vi "SetPwrSupAutomatic_v2.vi"(8 "error in (no error)":errorcluster, 10 "Enum":T1=enum."Control Power", 11 "HMP VISA":refnum<visa-resource-name>) -> (0 "error out":errorcluster, 3 "HMP VISA Out":refnum<visa-resource-name> caption="VISA resource name out")   [LabVIEW 2022 SP3]
doc: "This VI will command the Power Supply. Add enumerators and cases if new commands are needed"
uses:
  HMP4000 Communication/HMP4040_ChannelControlAutomatic.ctl
  HMP4000 Communication/HMP4040_ChannelControl.ctl
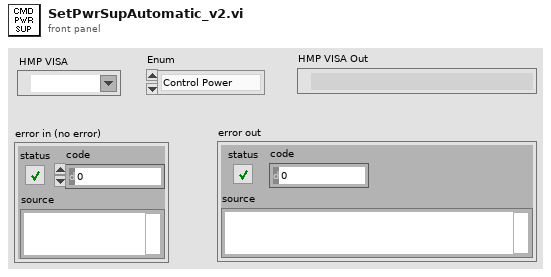
[diagram p1: front panel]
types:
  T1 = typedef "HMP4040_ChannelControlAutomatic.ctl" = enum16{"Off", "Control Power", "HMP2020 Control + DC32V", "HMP2020 Control + DC8V", "HMP4040 Control + DC32V", "HMP4040 Control +DC8V", "HMP4040 Ch2 24V 4A"}
  T2 = typedef "HMP4040_ChannelControl.ctl" = cluster{"CH1 Voltage":dbl, "CH1 Current":dbl, "CH1 Output":bool, "CH2 Voltage":dbl, "CH2 Current":dbl, "CH2 Output":bool, "CH3 Voltage":dbl, "CH3 Current":dbl, "CH3 Output":bool, "CH4 Voltage":dbl, "CH4 Current":dbl, "CH4 Output":bool, "Master Output":bool}
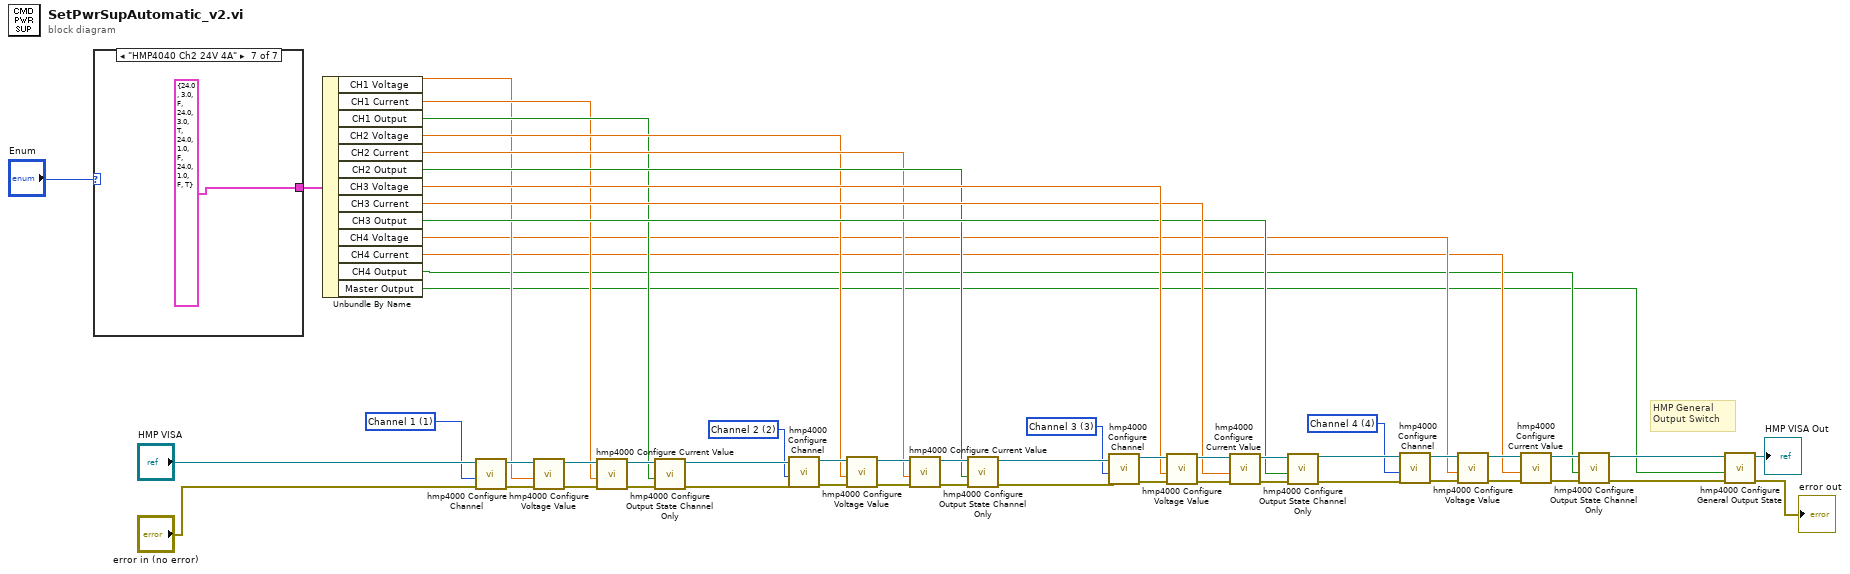
[diagram p0: block diagram]
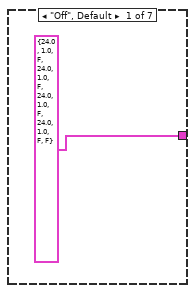
[diagram p2: hidden frame]
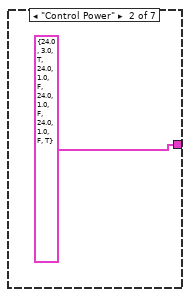
[diagram p3: hidden frame]
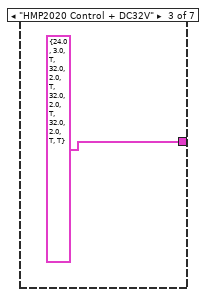
[diagram p4: hidden frame]
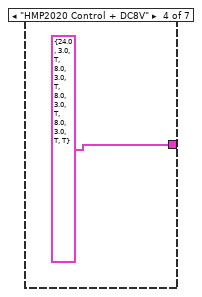
[diagram p5: hidden frame]
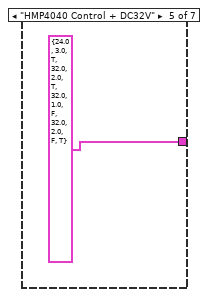
[diagram p6: hidden frame]
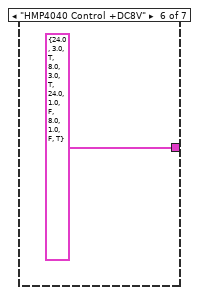
[diagram p7: hidden frame]
diagram:
  w16 = 4 items=["Channel 1"=1, "Channel 2"=2, "Channel 3"=3, "Channel 4"=4] ("Channel (Channel 1)")
  w15 = 3 items=["Channel 1"=1, "Channel 2"=2, "Channel 3"=3, "Channel 4"=4] ("Channel (Channel 1)")
  w14 = 2 items=["Channel 1"=1, "Channel 2"=2, "Channel 3"=3, "Channel 4"=4] ("Channel (Channel 1)")
  w17 = 1 items=["Channel 1"=1, "Channel 2"=2, "Channel 3"=3, "Channel 4"=4] ("Channel (Channel 1)")
  # "HMP General\nOutput Switch"
  n1 = case shown="\"HMP4040 Ch2 24V 4A\"" "Enum" {
    tunnel: [T2 {"CH1 Voltage"=24.0, "CH1 Current"=1.0, "CH1 Output"=FALSE, "CH2 Voltage"=24.0, "CH2 Current"=1.0, "CH2 Output"=FALSE, "CH3 Voltage"=24.0, "CH3 Current"=1.0, "CH3 Output"=FALSE, "CH4 Voltage"=24.0, "CH4 Current"=1.0, "CH4 Output"=FALSE, "Master Output"=FALSE} ("HMP4040 Channel Settings") T2 {"CH1 Voltage"=24.0, "CH1 Current"=3.0, "CH1 Output"=TRUE, "CH2 Voltage"=24.0, "CH2 Current"=1.0, "CH2 Output"=FALSE, "CH3 Voltage"=24.0, "CH3 Current"=1.0, "CH3 Output"=FALSE, "CH4 Voltage"=24.0, "CH4 Current"=1.0, "CH4 Output"=FALSE, "Master Output"=TRUE} ("HMP4040 Channel Settings") T2 {"CH1 Voltage"=24.0, "CH1 Current"=3.0, "CH1 Output"=TRUE, "CH2 Voltage"=32.0, "CH2 Current"=2.0, "CH2 Output"=TRUE, "CH3 Voltage"=32.0, "CH3 Current"=2.0, "CH3 Output"=TRUE, "CH4 Voltage"=32.0, "CH4 Current"=2.0, "CH4 Output"=TRUE, "Master Output"=TRUE} ("HMP4040 Channel Settings") T2 {"CH1 Voltage"=24.0, "CH1 Current"=3.0, "CH1 Output"=TRUE, "CH2 Voltage"=8.0, "CH2 Current"=3.0, "CH2 Output"=TRUE, "CH3 Voltage"=8.0, "CH3 Current"=3.0, "CH3 Output"=TRUE, "CH4 Voltage"=8.0, "CH4 Current"=3.0, "CH4 Output"=TRUE, "Master Output"=TRUE} ("HMP4040 Channel Settings") T2 {"CH1 Voltage"=24.0, "CH1 Current"=3.0, "CH1 Output"=TRUE, "CH2 Voltage"=32.0, "CH2 Current"=2.0, "CH2 Output"=TRUE, "CH3 Voltage"=32.0, "CH3 Current"=1.0, "CH3 Output"=FALSE, "CH4 Voltage"=32.0, "CH4 Current"=2.0, "CH4 Output"=FALSE, "Master Output"=TRUE} ("HMP4040 Channel Settings") T2 {"CH1 Voltage"=24.0, "CH1 Current"=3.0, "CH1 Output"=TRUE, "CH2 Voltage"=8.0, "CH2 Current"=3.0, "CH2 Output"=TRUE, "CH3 Voltage"=24.0, "CH3 Current"=1.0, "CH3 Output"=FALSE, "CH4 Voltage"=8.0, "CH4 Current"=1.0, "CH4 Output"=FALSE, "Master Output"=TRUE} ("HMP4040 Channel Settings") T2 {"CH1 Voltage"=24.0, "CH1 Current"=3.0, "CH1 Output"=FALSE, "CH2 Voltage"=24.0, "CH2 Current"=3.0, "CH2 Output"=TRUE, "CH3 Voltage"=24.0, "CH3 Current"=1.0, "CH3 Output"=FALSE, "CH4 Voltage"=24.0, "CH4 Current"=1.0, "CH4 Output"=FALSE, "Master Output"=TRUE} ("HMP4040 Channel Settings")] -> w46
    frame "Off", Default {
    }
    frame "Control Power" {
    }
    frame "HMP2020 Control + DC32V" {
    }
    frame "HMP2020 Control + DC8V" {
    }
    frame "HMP4040 Control + DC32V" {
    }
    frame "HMP4040 Control +DC8V" {
    }
    frame "HMP4040 Ch2 24V 4A" {
    }
  }
  n2 = Unbundle By Name(w46) -> ("CH1 Voltage"=w7:dbl, "CH1 Current"=w8:dbl, "CH1 Output"=w9:bool, "CH2 Voltage"=w10:dbl, "CH2 Current"=w11:dbl, "CH2 Output"=w12:bool, "CH3 Voltage"=w19:dbl, "CH3 Current"=w18:dbl, "CH3 Output"=w13:bool, "CH4 Voltage"=w6:dbl, "CH4 Current"=w5:dbl, "CH4 Output"=w4:bool, "Master Output"=w3:bool)
  n3 = call <instrlib>:"hmp4000 Configure Channel.vi"("error in (no error)"="error in (no error)", "Channel (Channel 1)"=w17, "VISA resource name"="HMP VISA") -> ("error out"=w52:errorcluster, "VISA resource name out"=w51:refnum<visa-resource-name>)  [unwired: 7 in]
  n4 = call <instrlib>:"hmp4000 Configure Voltage Value.vi"("error in (no error)"=w52, "Voltage (0.0)"=w7, "VISA resource name"=w51) -> ("error out"=w50:errorcluster, "VISA resource name out"=w49:refnum<visa-resource-name>)  [unwired: 7 in]
  n5 = call <instrlib>:"hmp4000 Configure Current Value.vi"("error in (no error)"=w50, "Current (0.0)"=w8, "VISA resource name"=w49) -> ("error out"=w48:errorcluster, "VISA resource name out"=w47:refnum<visa-resource-name>)  [unwired: 7 in]
  n6 = call <instrlib>:"hmp4000 Configure Output State Channel Only.vi"("error in (no error)"=w48, "Output State (Off)"=w9, "VISA resource name"=w47) -> ("error out"=w26:errorcluster, "VISA resource name out"=w27:refnum<visa-resource-name>)  [unwired: 7 in]
  n7 = call <instrlib>:"hmp4000 Configure Channel.vi"("error in (no error)"=w26, "Channel (Channel 1)"=w14, "VISA resource name"=w27) -> ("error out"=w40:errorcluster, "VISA resource name out"=w41:refnum<visa-resource-name>)  [unwired: 7 in]
  n8 = call <instrlib>:"hmp4000 Configure Voltage Value.vi"("error in (no error)"=w40, "Voltage (0.0)"=w10, "VISA resource name"=w41) -> ("error out"=w42:errorcluster, "VISA resource name out"=w43:refnum<visa-resource-name>)  [unwired: 7 in]
  n9 = call <instrlib>:"hmp4000 Configure Current Value.vi"("error in (no error)"=w42, "Current (0.0)"=w11, "VISA resource name"=w43) -> ("error out"=w44:errorcluster, "VISA resource name out"=w45:refnum<visa-resource-name>)  [unwired: 7 in]
  n10 = call <instrlib>:"hmp4000 Configure Output State Channel Only.vi"("error in (no error)"=w44, "Output State (Off)"=w12, "VISA resource name"=w45) -> ("error out"=w24:errorcluster, "VISA resource name out"=w25:refnum<visa-resource-name>)  [unwired: 7 in]
  n11 = call <instrlib>:"hmp4000 Configure Channel.vi"("error in (no error)"=w24, "Channel (Channel 1)"=w15, "VISA resource name"=w25) -> ("error out"=w39:errorcluster, "VISA resource name out"=w38:refnum<visa-resource-name>)  [unwired: 7 in]
  n12 = call <instrlib>:"hmp4000 Configure Voltage Value.vi"("error in (no error)"=w39, "Voltage (0.0)"=w19, "VISA resource name"=w38) -> ("error out"=w37:errorcluster, "VISA resource name out"=w36:refnum<visa-resource-name>)  [unwired: 7 in]
  n13 = call <instrlib>:"hmp4000 Configure Current Value.vi"("error in (no error)"=w37, "Current (0.0)"=w18, "VISA resource name"=w36) -> ("error out"=w35:errorcluster, "VISA resource name out"=w34:refnum<visa-resource-name>)  [unwired: 7 in]
  n14 = call <instrlib>:"hmp4000 Configure Output State Channel Only.vi"("error in (no error)"=w35, "Output State (Off)"=w13, "VISA resource name"=w34) -> ("error out"=w23:errorcluster, "VISA resource name out"=w22:refnum<visa-resource-name>)  [unwired: 7 in]
  n15 = call <instrlib>:"hmp4000 Configure Channel.vi"("error in (no error)"=w23, "Channel (Channel 1)"=w16, "VISA resource name"=w22) -> ("error out"=w28:errorcluster, "VISA resource name out"=w29:refnum<visa-resource-name>)  [unwired: 7 in]
  n16 = call <instrlib>:"hmp4000 Configure Voltage Value.vi"("error in (no error)"=w28, "Voltage (0.0)"=w6, "VISA resource name"=w29) -> ("error out"=w30:errorcluster, "VISA resource name out"=w31:refnum<visa-resource-name>)  [unwired: 7 in]
  n17 = call <instrlib>:"hmp4000 Configure Current Value.vi"("error in (no error)"=w30, "Current (0.0)"=w5, "VISA resource name"=w31) -> ("error out"=w32:errorcluster, "VISA resource name out"=w33:refnum<visa-resource-name>)  [unwired: 7 in]
  n18 = call <instrlib>:"hmp4000 Configure Output State Channel Only.vi"("error in (no error)"=w32, "Output State (Off)"=w4, "VISA resource name"=w33) -> ("error out"=w20:errorcluster, "VISA resource name out"=w21:refnum<visa-resource-name>)  [unwired: 7 in]
  n19 = call <instrlib>:"hmp4000 Configure General Output State.vi"("error in (no error)"=w20, "Output State (Off)"=w3, "VISA resource name"=w21) -> ("error out"=→"error out":errorcluster, "VISA resource name out"=→"HMP VISA Out":refnum<visa-resource-name>)  [unwired: 7 in]
